vi "api-example.control-digital-output.vi"(10 "Baud Rate":u32(ring)=57600 items=["75"=75, "110"=110, "134"=134, "150"=150, "300"=300, "600"=600, "1200"=1200, "1800"=1800, "2400"=2400, "4800"=4800, "7200"=7200, "9600"=9600, "14400"=14400, "19200"=19200, "28800"=28800, "38400"=38400, "56000"=56000, "57600"=57600, "115200"=115200, "128000"=128000, "230400"=230400], 11 "Comport":refnum<visa-resource-name>="COM20") -> (0 "error out":errorcluster)   [LabVIEW 2020]
doc: "Example showing the use of the api to control a digital line"
uses:
  FirmataClient/Controls/FirmataPinCapabilitiesAndAnalogMapping.ctl
  FirmataClient/Controls/FirmataPinCapability.ctl
  FirmataClient/Controls/FirmataPinModes.ctl
  FirmataClient/FirmataClient.lvlib
panel:
  in  "Tab Control":enum32{"Connection", "Example"}(tab)
  in  "Connection Details":enum32{"Serial Communication"}(tab)
  out "Firmata Firmware Version":string
  out "Firmata Firmware Name":string
  in  "Query Capabilities?":bool
  out "Connected":bool
  in  "Pin Index":u8=13
  out "Pin Value Out":bool
  in  "Stop":bool
  out "Board Capabilities":map{i32, T1}(c390)
  # "Toggling Pin below every 500ms"
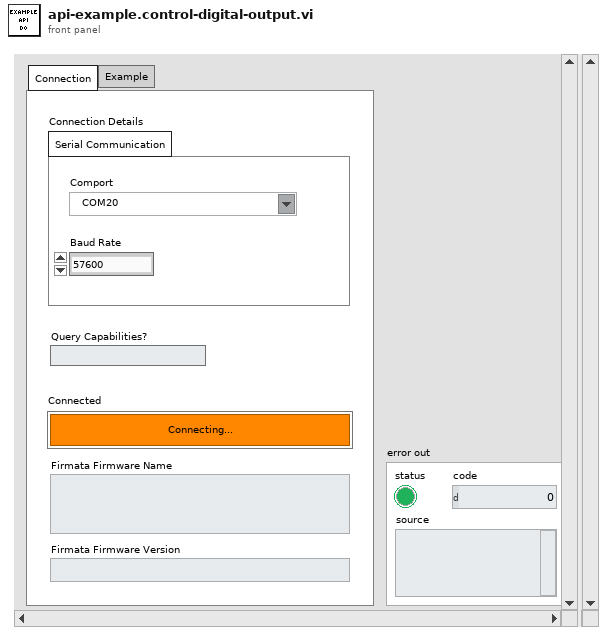
[diagram p1: front panel]
types:
  T1 = typedef "FirmataClient.lvlib/FirmataPinCapabilitiesAndAnalogMapping.ctl" = cluster{"Supported Modes":T2[], "Analog Channel":u8, "Pin Name":string}
  T2 = typedef "FirmataClient.lvlib/FirmataPinCapability.ctl" = cluster{"PinMode":T3, "Resolution":u8}
  T3 = typedef "FirmataClient.lvlib/FirmataPinModes.ctl" = enum16{"DigitalInput", "DigitalOutput", "AnalogInput", "PWM", "Servo", "Shift", "I2C", "OneWire", "Stepper", "Encoder", "Serial", "InputPullup", "Extended.SPI", "Extended.Sonar", "Extended.Tone", "Extended.DHT"}
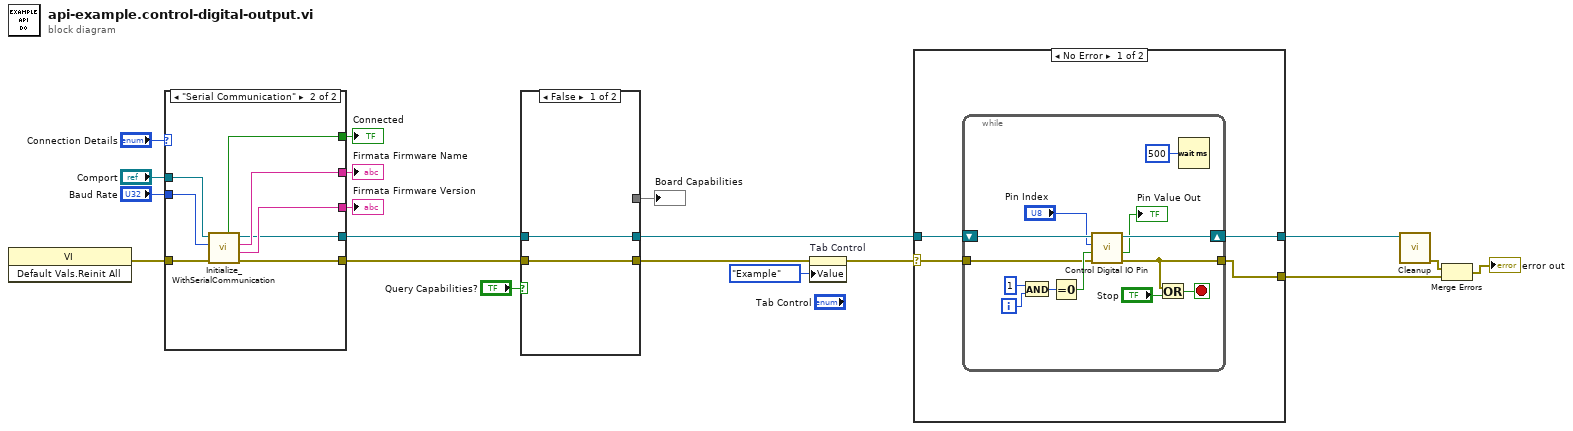
[diagram p0: block diagram]
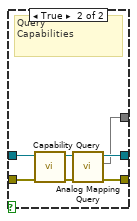
[diagram p3: hidden frame]
diagram:
  n1 = invoke class="VI" method="Default Vals.Reinit All"() -> (error out=w17:errorcluster)  [unwired: 3 in, 2 out]
  n2 = case shown="\"Serial Communication\"" "Connection Details" {
    tunnel: w17 -> [w20 w28]
    tunnel: "Baud Rate" -> [_ w27]
    tunnel: "Comport" -> [_ w26]
    tunnel: [_ w25] -> w14
    tunnel: [_ w24] -> w13
    tunnel: [_ w23] -> w10
    tunnel: [w20 w22] -> w9
    tunnel: [_ w21] -> w2
    frame Default {
    }
    frame "Serial Communication" {
      n3 = call "Initialize_WithSerialCommunication.vi"("error in"=w28, "Baud Rate"=w27, "Comport"=w26) -> ("error out"=w22:errorcluster, "FirmataFirmwareVersion"=w24:string, "FirmataFirmwareName"=w25:string, "Refnum Out"=w23:refnum<vi>, "Connected"=w21:bool)  [unwired: 4 in]
    }
  }
  "Firmata Firmware Name" <- w14
  "Firmata Firmware Version" <- w13
  "Connected" <- w2
  n4 = case shown="False" "Query Capabilities?" {
    tunnel: w10 -> [w30 w37]
    tunnel: w9 -> [w29 w36]
    tunnel: [w30 w33] -> w8
    tunnel: [w29 w32] -> w4
    tunnel: [_ w31] -> w6
    frame False {
    }
    frame True {
      # "Query \nCapabilities"
      n5 = call "Capability Query.vi"("error in (no error)"=w36, "Refnum In"=w37) -> ("error out"=w34:errorcluster, "Refnum Out"=w35:refnum<vi>)  [unwired: 7 in, 1 out]
      n6 = call "Analog Mapping Query.vi"("error in (no error)"=w34, "Refnum In"=w35) -> ("error out"=w32:errorcluster, "Board Capabilities"=w31:map{i32, T1}, "Refnum Out"=w33:refnum<vi>)  [unwired: 7 in]
    }
  }
  "Board Capabilities" <- w6
  n7 = property on="Tab Control" class="TabCtl (strict)"(error in=w4, "Value"=enum32{"Connection", "Example"}."Example" ("Tab Control")) -> (error out=w3:errorcluster)  [unwired: 1 in, 1 out]
  n8 = case shown="No Error" w3 {
    selector: w3 -> [w39 w55]
    tunnel: [w38 w55] -> w12
    tunnel: [w41 w56] -> w11
    tunnel: w8 -> [w40 w56]
    frame No Error {
      n9 = while {
        shift-right: [w53] -> w41
        shift-left: w40 -> [w54]
        tunnel: w39 -> [w45]
        tunnel: [w44] -> w38
        i -> [w51]
        stop <- w42 stop-if-true
        n10 = And(x=1, y=w51) -> (x .and. y?=w49:i32)
        n11 = Equal To 0?(x=w49) -> (x = 0?=w48:bool)
        n12 = call "Control Digital IO Pin.vi"("error in (no error)"=w45, "Pin Value"=w48, "Pin Index"="Pin Index", "Refnum In"=w54) -> ("error out"=w44:errorcluster, "Pin Value Out"=→"Pin Value Out":bool, "Refnum Out"=w53:refnum<vi>)  [unwired: 4 in, 1 out]
        n13 = Or(x=w44, y="Stop") -> (x .or. y?=w42:bool)
        n14 = Wait (ms)(milliseconds to wait=u32 500) -> ()  [unwired: 1 out]
      }
    }
    frame Error {
    }
  }
  n15 = call "Cleanup.vi"("Refnum In"=w11) -> ("error out"=w19:errorcluster)  [unwired: 10 in]
  n16 = Merge Errors(w19, w12) -> (→"error out":errorcluster)
